vi "SoftFrontPanel.vi"(11 "Thermo Instrument":refnum<class "Thermo Instrument.lvclass">) -> ()   [LabVIEW 2025, in "Thermo.lvlib" / "Thermo Instrument.lvclass"]
doc: "Copyright 2017 National Instruments Corporation\n\nLicensed under the Apache License, Version 2.0 (the \"License\"); you may not use this file except in compliance with the License. You may obtain a copy of the License at http://www.apache.org/licenses/LICENSE-2.0\nUnless required by applicable law or agreed to in writing, software distributed under the License is distributed on an \"AS IS\" BASIS, WITHOUT WARRANTIES OR CONDITIONS OF ANY KIND, either express or implied. See the License for the specific language governing permissions and limitations under the License."
uses:
  Thermo Instrument.lvclass
  Thermo Instrument.lvclass/Thermo Instrument.ctl
  Thermo configuration/Thermo configuration.lvclass
panel:
  out "Channels":T1(array[cluster]) {"Measurement" format="%#_4p"}
  out "Instrument":string caption="Instrument ::"
  # "ch"
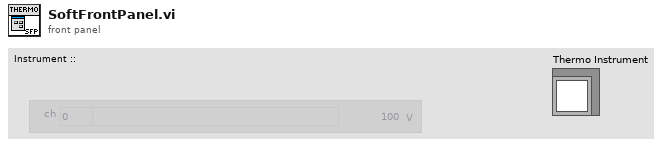
[diagram p1: front panel]
types:
  T1 = cluster{"Channel Alias":string, "Index":i32, "Measurement":dbl}[]
  T2 = enum32{"Invalid", "Default", "Floating", "Floating/Auto-Hide", "Modal"}
  T3 = typedef "Abstract Engine.lvlibp/Instrument configuration.lvclass/Default Instrument.ctl" = cluster{"Type":string, "Address":string, "SW Alias":string, "Description":string, "Enabled":bool}
  T4 = cluster{"Channel Alias":string, "Index":i32, "Measurement":dbl}
  T5 = cluster{"Alias":string, "DataType":enum16{"Anaolg Input", "Waveform"}, "Unit":enum16{"---", "V", "A", "Ohm", "Hz", "uF", "degC", "deg"}, "Upper limit":dbl, "Lower limit":dbl, "Measurement":variant}[]
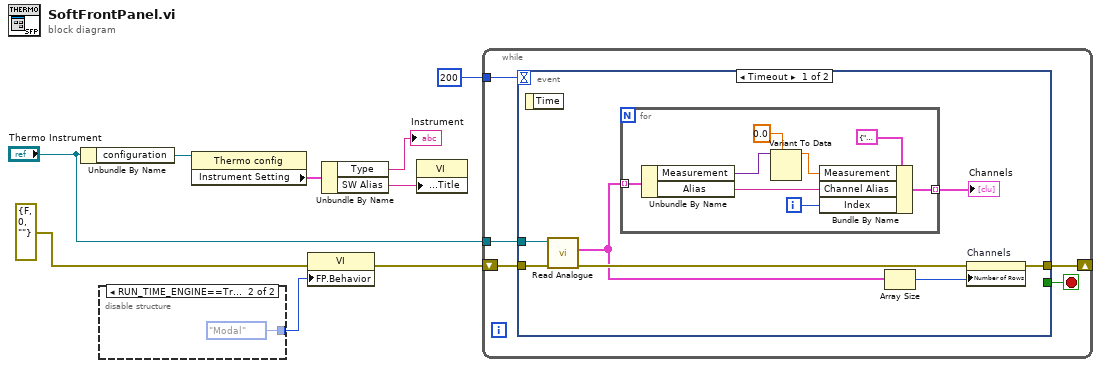
[diagram p0: block diagram]
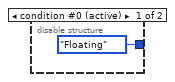
[diagram p2: hidden frame]
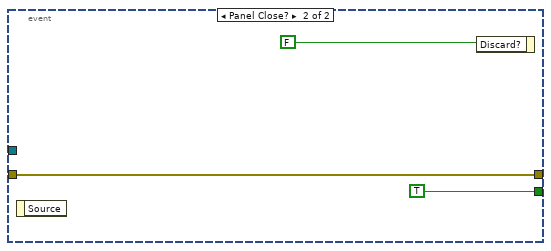
[diagram p3: hidden frame]
diagram:
  n1 = Unbundle By Name("Thermo Instrument") -> ("configuration"=w5:refnum<class "Thermo configuration.lvclass">)
  n2 = disable-structure shown="RUN_TIME_ENGINE==True" {
    disable-tunnel: [T2."Floating" ("Front Panel Window:Behavior") T2."Modal" ("Front Panel Window:Behavior")] -> w8
    frame condition #0 (active) {
    }
    frame condition #1 {
    }
  }
  n3 = property class="Thermo config"(reference=w5) -> ("Instrument Setting"=w4:T3)  [unwired: 1 in, 2 out]
  n4 = property class="VI"(error in=errorcluster {"status"=FALSE, "code"=0, "source"=""} ("error in (no error)"), "FP.Behavior"=w8) -> (error out=w7:errorcluster)  [unwired: 1 in, 1 out]
  n5 = Unbundle By Name(w4) -> ("Type"=→"Instrument":string, "SW Alias"=w3:string)
  n6 = property class="VI"("Front Panel.Title"=w3) -> ()  [unwired: 2 in, 2 out]
  n7 = while {
    shift-right: [w14] -> _
    shift-left: w7 -> [w15]
    tunnel: 200 -> [w12]
    tunnel: "Thermo Instrument" -> [w13]
    stop <- w16 stop-if-true
    n8 = event shown="[0] Timeout" {
      selector: _ -> [_ _]
      dyn-events: _ -> [_ _]
      timeout: w12 -> [_ _]
      tunnel: [_ TRUE] -> w16
      tunnel: [w19 w32] -> w14
      tunnel: w15 -> [w22 w32]
      tunnel: w13 -> [w23 _]
      event Timeout {
        n9 = event-data() -> ()  [unwired: 1 in, 1 out]
        n10 = call-dynamic "Read Analogue.vi"("error in (no error)"=w22, "Analog Input in"=w23) -> ("error out"=w18:errorcluster, "Measurements"=w17:T5)  [unwired: 7 in, 1 out]
        n11 = for {
          tunnel: [w29] -> w21 mode=indexing
          tunnel: w17 -> [w28] mode=indexing
          i -> [w30]
          n12 = Unbundle By Name(w28) -> ("Measurement"=w26:variant, "Alias"=w27:string)
          n13 = Variant To Data(type=0.0 ("Measurement"), Variant=w26) -> (data=w24:dbl)  [unwired: 1 in, 1 out]
          n14 = Bundle By Name(cluster=T4 {"Channel Alias"="", "Index"=0, "Measurement"=100.0} ("Channel"), "Measurement"=w24, "Channel Alias"=w27, "Index"=w30) -> (w29:T4)
        }
        "Channels" <- w21
        n15 = Array Size(array=w17) -> (size(s)=w20:i32)
        n16 = property on="Channels" class="Arr (strict)"(error in=w18, "Number of Rows"=w20) -> (error out=w19:errorcluster)  [unwired: 1 in, 1 out]
      }
      event Panel Close? {
        n17 = event-data() -> ()  [unwired: 1 in, 1 out]
        n18 = event-data("Discard?"=FALSE) -> ()  [unwired: 1 in, 1 out]
      }
    }
  }
